vi "Facade.vi"(0 "Data In":T5, 2 "Display State In":T2={"Prompt"="Click to add", "Listbox"=refnum, "events"={"Items Changed"=refnum, "List Changed"=refnum}, "allow move"=FALSE}, 3 "Container State":T4) -> (6 "Data Out":T5, 7 "Display State Out":T2={"Prompt"="Click to add", "Listbox"=refnum, "events"={"Items Changed"=refnum, "List Changed"=refnum}, "allow move"=FALSE}, 8 "Action":T1)   [LabVIEW 2020, in "KListbox.xctl"]
uses:
  KListbox.xctl
  Data.ctl
  <vilib>/_xctls/Container State.ctl
  State.ctl
  Events.ctl
  Event Action.ctl
  <vilib>/_xctls/Action.ctl
  <vilib>/_xctls/XControlSupport.lvlib
panel:
  out "drag from":i32
  in  "Listbox":i32(listbox)
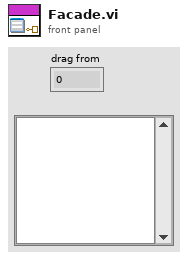
[diagram p1: front panel]
types:
  T1 = typedef "XControlSupport.lvlib/Action.ctl" = cluster{"Data Changed?":bool, "State Changed?":bool, "Action Name":string}
  T2 = typedef "KListbox.xctl/State.ctl" = cluster{"Prompt":string, "Listbox":refnum<vi>, "events":T3, "allow move":bool}
  T3 = typedef "KListbox.xctl/Events.ctl" = cluster{"Items Changed":refnum<user-event>, "List Changed":refnum<user-event>}
  T4 = typedef "XControlSupport.lvlib/Container State.ctl" = cluster{"Indicator?":bool, "Run Mode?":bool, " Refnum":refnum<vi>}
  T5 = typedef "KListbox.xctl/Data.ctl" = cluster{"Row":i32, "Items":string[]}
  T6 = typedef "KListbox.xctl/Event Action.ctl" = enum16{"Select", "Add", "Delete", "Edit"}
  T7 = typedef "LVPoint32TypeDef.ctl" = cluster{"Horizontal":i32, "Vertical":i32}
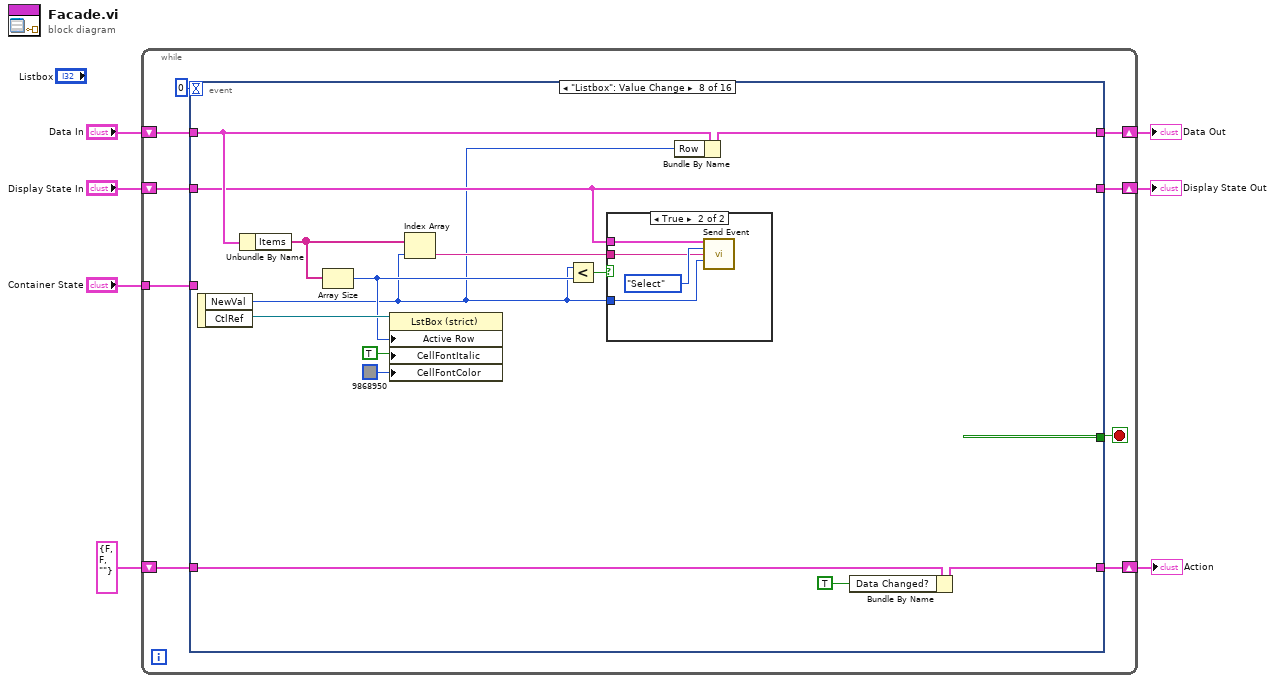
[diagram p0: block diagram]
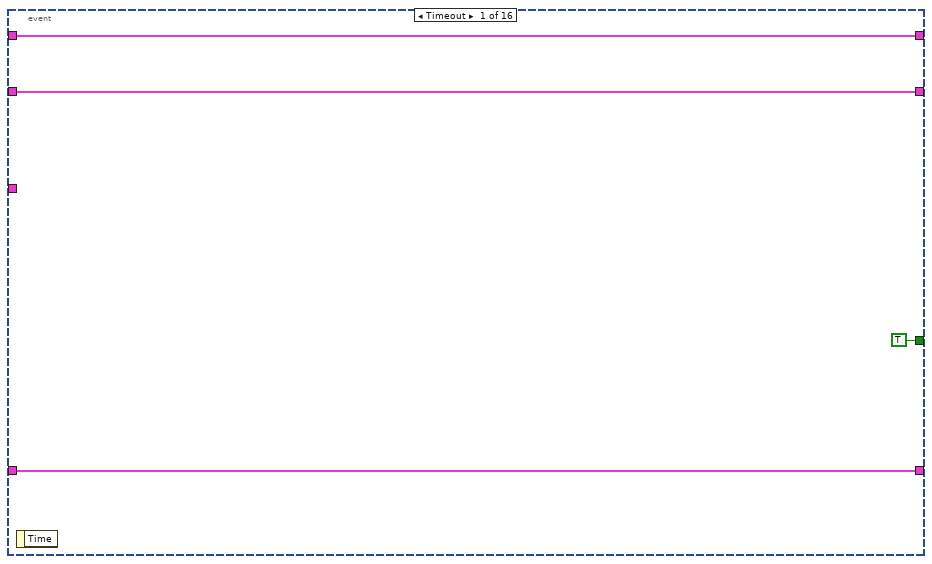
[diagram p2: hidden frame]
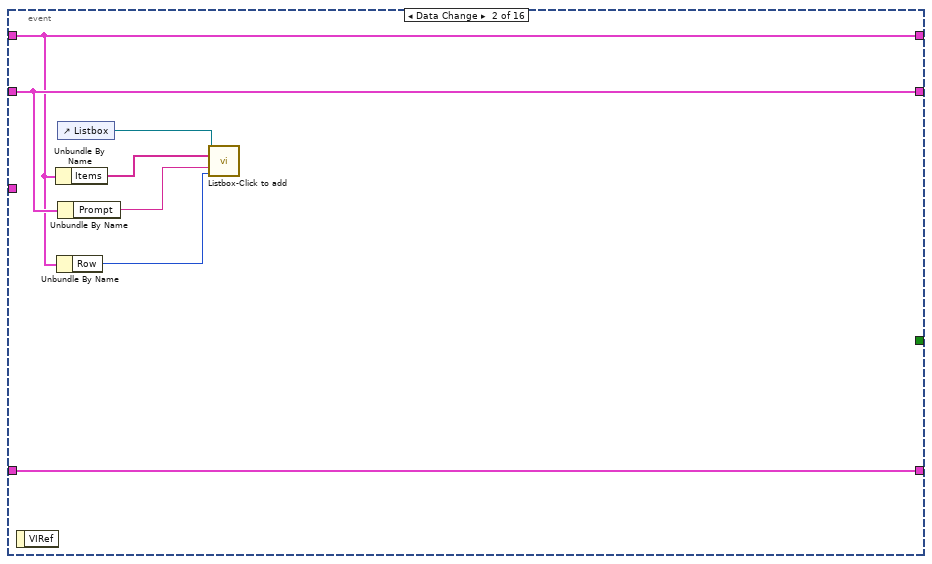
[diagram p3: hidden frame]
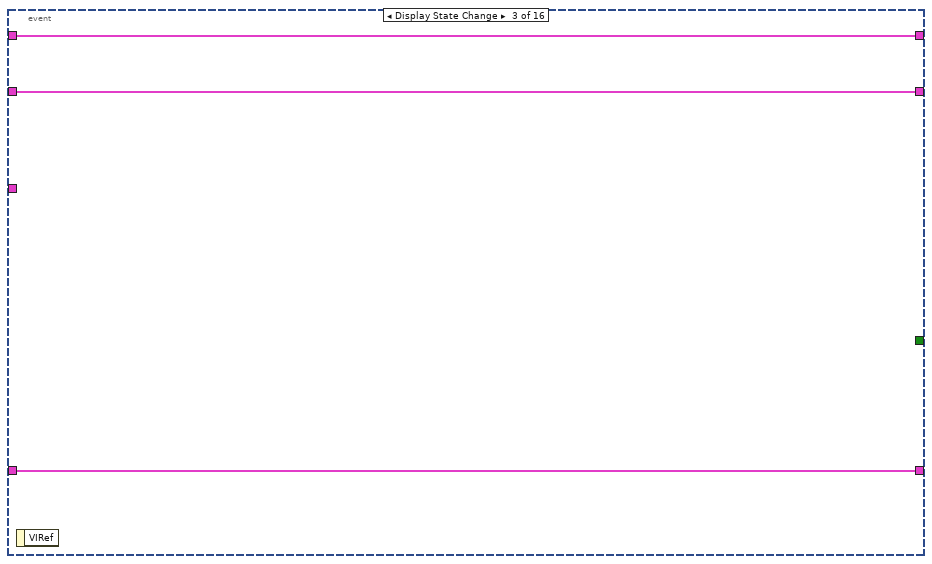
[diagram p4: hidden frame]
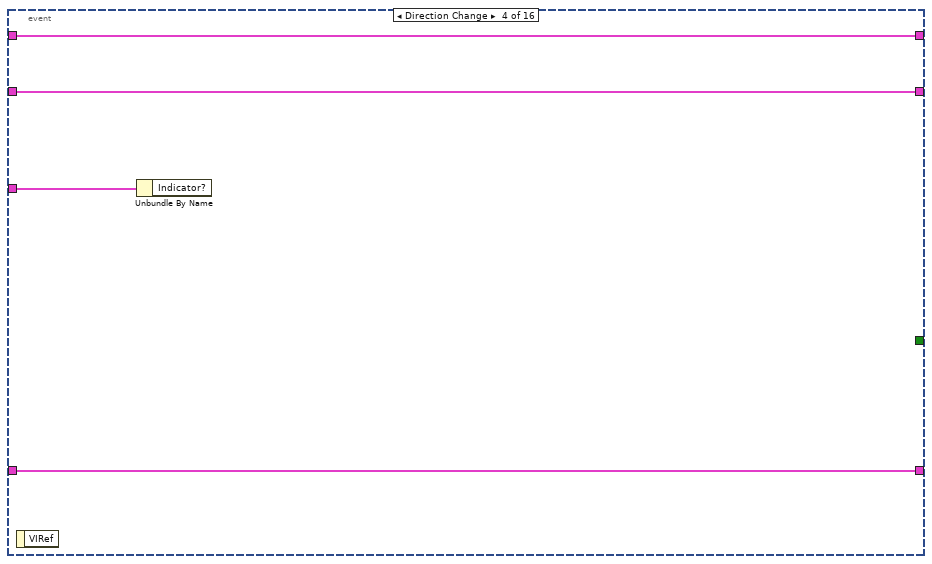
[diagram p5: hidden frame]
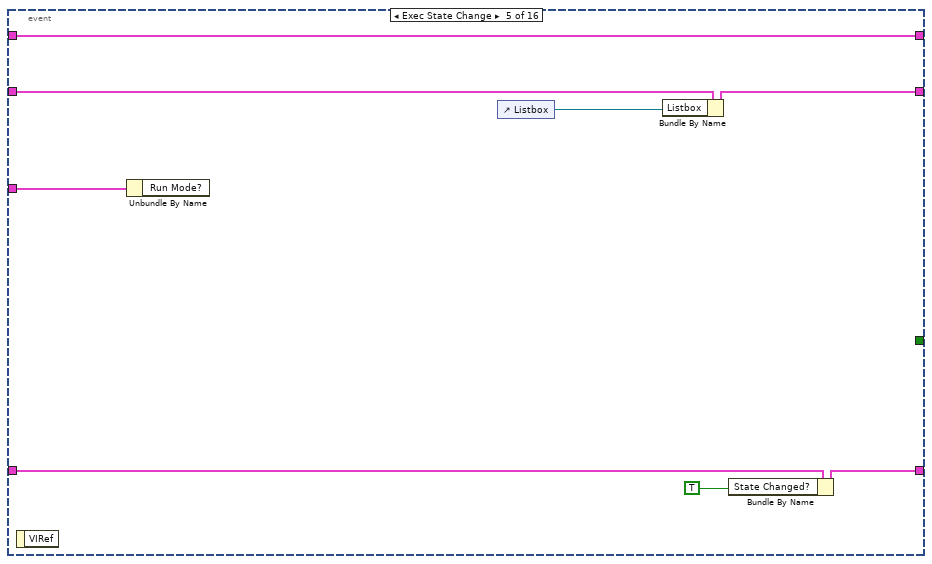
[diagram p6: hidden frame]
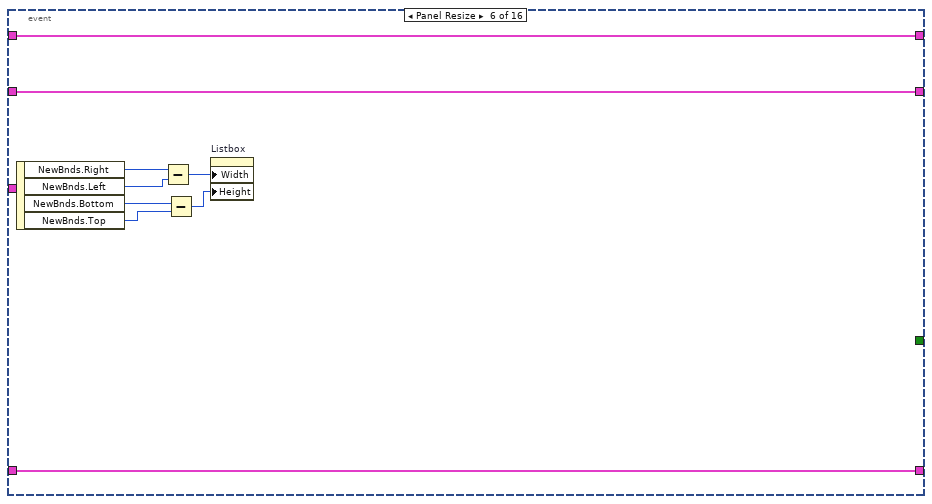
[diagram p7: hidden frame]
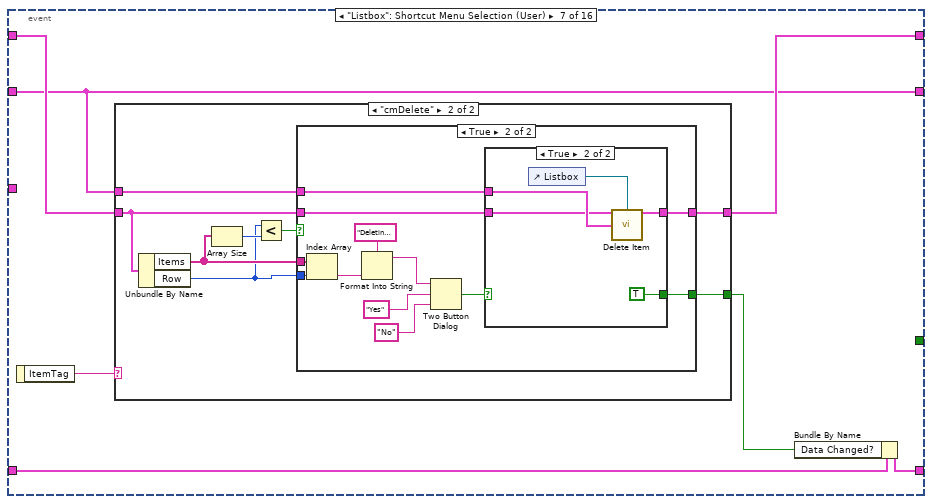
[diagram p8: hidden frame]
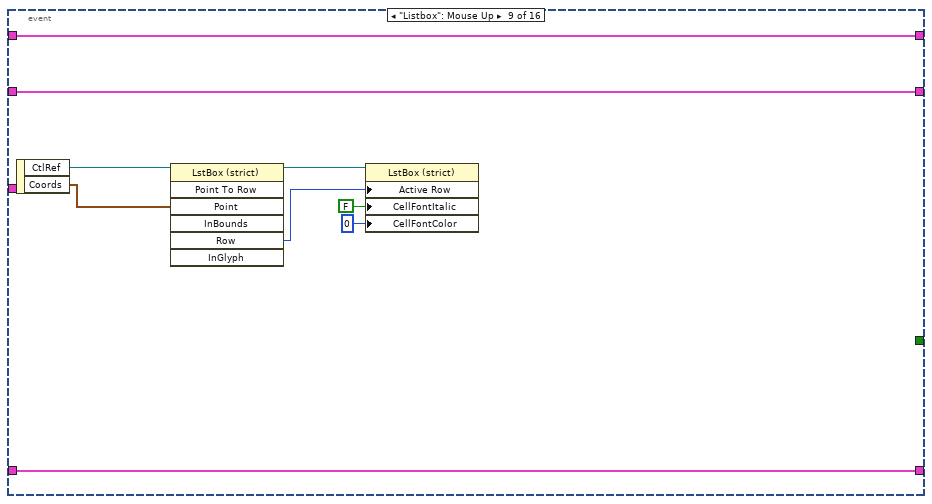
[diagram p13: hidden frame]
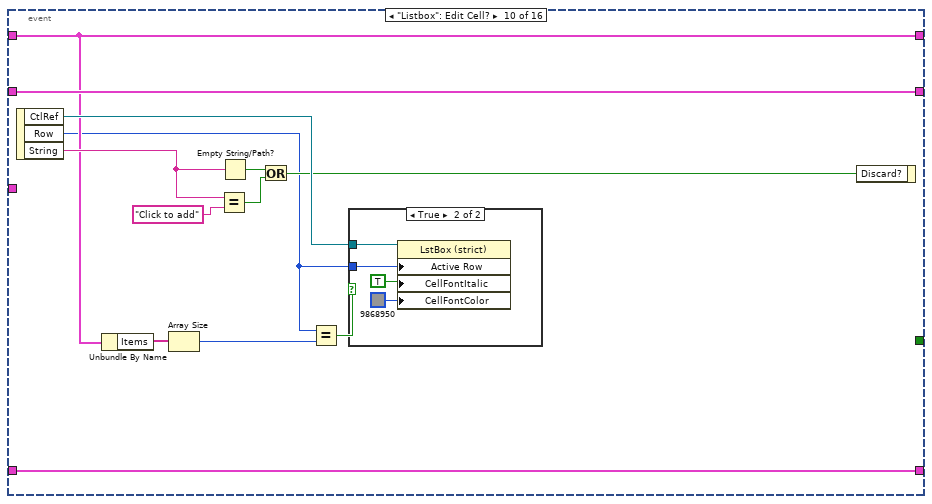
[diagram p14: hidden frame]
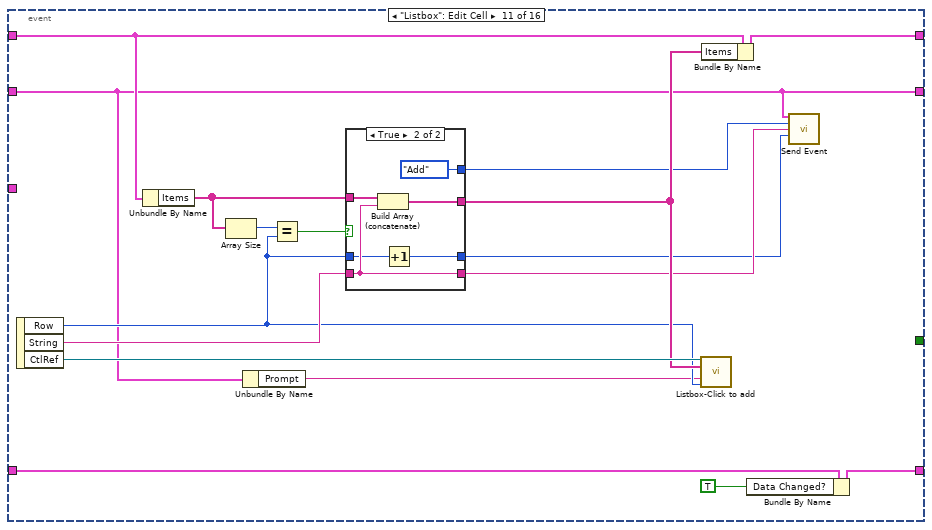
[diagram p16: hidden frame]
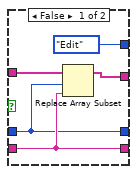
[diagram p17: hidden frame]
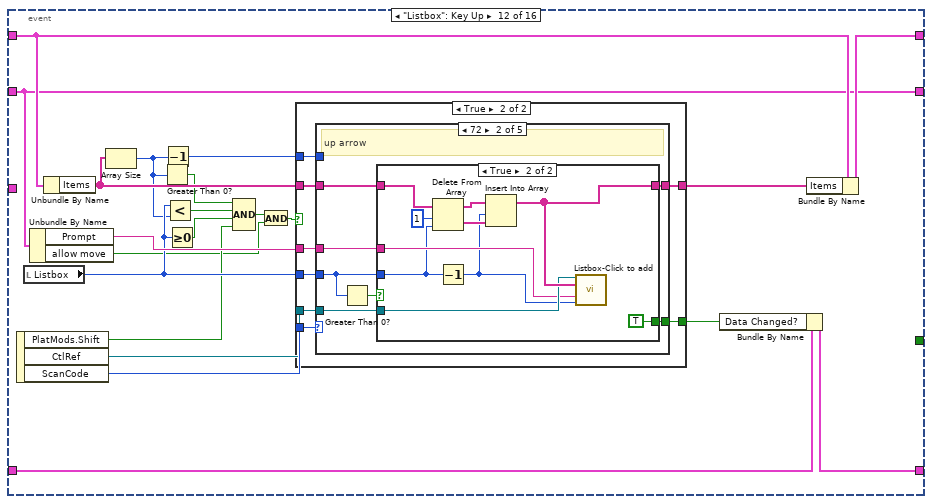
[diagram p18: hidden frame]
diagram:
  n1 = while {
    shift-right: [w15] -> w4
    shift-left: "Display State In" -> [w16]
    tunnel: "Container State" -> [w12]
    shift-right: [w10] -> w7
    shift-left: "Data In" -> [w11]
    shift-right: [w8] -> w2
    shift-left: T1 {"Data Changed?"=FALSE, "State Changed?"=FALSE, "Action Name"=""} ("Action") -> [w9]
    stop <- w14 stop-if-true
    n2 = event shown="[7] \"Listbox\": Value Change" {
      selector: _ -> [_ _ _ _ _ _ _ _ _ _ _ _ _ _ _ _]
      dyn-events: _ -> [_ _ _ _ _ _ _ _ _ _ _ _ _ _ _ _]
      timeout: 0 -> [_ _ _ _ _ _ _ _ _ _ _ _ _ _ _ _]
      tunnel: w16 -> [w18 w26 w30 w33 w41 w51 w53 w92 w113 w126 w134 w171 w251 w255 w265 w268]
      tunnel: [w18 w26 w30 w33 w38 w51 w53 w92 w113 w126 w134 w171 w251 w255 w265 w268] -> w15
      tunnel: [TRUE _ _ _ _ _ _ _ _ _ _ _ _ _ _ _] -> w14
      tunnel: w12 -> [_ _ _ w34 w42 _ _ _ _ _ _ _ _ _ _ _]
      tunnel: w11 -> [w17 w25 w29 w32 w40 w50 w55 w99 w112 w118 w146 w174 w250 w256 w264 w277]
      tunnel: [w17 w25 w29 w32 w40 w50 w54 w95 w112 w118 w141 w173 w250 w256 w264 w274] -> w10
      tunnel: [w19 w27 w28 w31 w36 w49 w56 w94 w111 w125 w140 w178 w249 w261 w263 w272] -> w8
      tunnel: w9 -> [w19 w27 w28 w31 w39 w49 w58 w100 w111 w125 w147 w179 w249 w261 w263 w278]
      event Timeout {
        n3 = event-data() -> ()  [unwired: 1 in, 1 out]
      }
      event Data Change {
        n4 = event-data() -> ()  [unwired: 1 in, 1 out]
        n5 = Unbundle By Name(w25) -> ("Items"=w23:string[])
        n6 = Unbundle By Name(w25) -> ("Row"=w21:i32)
        n7 = control-ref of="Listbox"() -> (w24:refnum<vi>)
        n8 = Unbundle By Name(w26) -> ("Prompt"=w22:string)
        n9 = call "Listbox-Click to add.vi"("ListBox"=w24, "Strings"=w23, "Prompt"=w22, "Row"=w21) -> ()  [unwired: 10 in, 2 out]
      }
      event Display State Change {
        n10 = event-data() -> ()  [unwired: 1 in, 1 out]
      }
      event Direction Change {
        n11 = event-data() -> ()  [unwired: 1 in, 1 out]
        n12 = Unbundle By Name(w34) -> ()  [unwired: 1 out]
      }
      event Exec State Change {
        n13 = event-data() -> ()  [unwired: 1 in, 1 out]
        n14 = Unbundle By Name(w42) -> ()  [unwired: 1 out]
        n15 = control-ref of="Listbox"() -> (w37:refnum<vi>)
        n16 = Bundle By Name(cluster=w41, "Listbox"=w37) -> (w38:T2)
        n17 = Bundle By Name(cluster=w39, "State Changed?"=TRUE) -> (w36:T1)
      }
      event Panel Resize {
        n18 = event-data() -> ("NewBnds.Right"=w48:i16, "NewBnds.Left"=w47:i16, "NewBnds.Bottom"=w46:i16, "NewBnds.Top"=w45:i16)  [unwired: 1 in]
        n19 = Subtract(x=w48, y=w47) -> (x-y=w44:i16)
        n20 = Subtract(x=w46, y=w45) -> (x-y=w43:i16)
        n21 = property on="Listbox" class="LstBox (strict)"("Width"=w44, "Height"=w43) -> ()  [unwired: 2 in, 2 out]
      }
      event "Listbox": Shortcut Menu Selection (User) {
        n22 = event-data() -> ("ItemTag"=w57:string)  [unwired: 1 in]
        n23 = case shown="\"cmDelete\"" w57 {
          tunnel: w55 -> [w59 w65]
          tunnel: [w59 w67] -> w54
          tunnel: w53 -> [_ w66]
          tunnel: [_ w60] -> w52
          frame "", Default {
          }
          frame "cmDelete" {
            n24 = Unbundle By Name(w65) -> ("Items"=w63:string[], "Row"=w62:i32)
            n25 = Array Size(array=w63) -> (size(s)=w64:i32)
            n26 = Less?(x=w62, y=w64) -> (x < y?=w61:bool)
            n27 = case shown="True" w61 {
              tunnel: [w68 w80] -> w67
              tunnel: w66 -> [_ w79]
              tunnel: w65 -> [w68 w78]
              tunnel: w63 -> [_ w71]
              tunnel: w62 -> [_ w70]
              tunnel: [_ w69] -> w60
              frame False {
              }
              frame True {
                n28 = Index Array(array=w71, index=w70) -> (element=w75:string)
                n29 = Format Into String(format string="Deleting '%s' cannot be undone. Are you sure you want to do it?", w75) -> (resulting string=w74:string)  [unwired: 2 in, 1 out]
                n30 = Two Button Dialog(message=w74, 1:"No" ("F button name (\"Cancel\")"), 2:"Yes" ("T button name (\"OK\")")) -> (T button?=w72:bool)
                n31 = case shown="True" w72 {
                  tunnel: [w81 w86] -> w80
                  tunnel: w79 -> [_ w85]
                  tunnel: w78 -> [w81 w84]
                  tunnel: [_ TRUE] -> w69
                  frame False {
                  }
                  frame True {
                    n32 = control-ref of="Listbox"() -> (w82:refnum<vi>)
                    n33 = call "Delete Item.vi"("Data In in"=w84, "LstBox Refnum"=w82, "Display State In"=w85) -> ("Data In out"=w86:T5)  [unwired: 12 in]
                  }
                }
              }
            }
          }
        }
        n34 = Bundle By Name(cluster=w58, "Data Changed?"=w52) -> (w56:T1)
      }
      event "Listbox": Value Change {
        n35 = event-data() -> ("NewVal"=w87:i32, "CtlRef"=w96:refnum<vi>)  [unwired: 1 in]
        n36 = Unbundle By Name(w99) -> ("Items"=w90:string[])
        n37 = Array Size(array=w90) -> (size(s)=w89:i32)
        n38 = property on="Property Node" class="LstBox (strict)"(reference=w96, "Active Row"=w89, "CellFontItalic"=TRUE ("Active Cell:Cell Font:Italic"), "CellFontColor"=u32 9868950) -> ()  [unwired: 1 in, 2 out]
        n39 = Index Array(array=w90, index=w87) -> (element=w88:string)
        n40 = Less?(x=w87, y=w89) -> (x < y?=w91:bool)
        n41 = case shown="True" w91 {
          tunnel: w92 -> [_ w104]
          tunnel: w87 -> [_ w102]
          tunnel: w88 -> [_ w101]
          frame False {
          }
          frame True {
            n42 = call "Send Event.vi"("State"=w104, "action"=Event_Action."Select", "Name"=w101, "Row"=w102) -> ()  [unwired: 10 in, 2 out]
          }
        }
        n43 = Bundle By Name(cluster=w99, "Row"=w87) -> (w95:T5)
        n44 = Bundle By Name(cluster=w100, "Data Changed?"=TRUE) -> (w94:T1)
      }
      event "Listbox": Mouse Up {
        n45 = event-data() -> ("CtlRef"=w106:refnum<vi>, "Coords"=w105:T7)  [unwired: 1 in]
        n46 = invoke on="Invoke Node" class="LstBox (strict)" method="Point To Row"(reference=w106, "Point"=w105) -> (reference out=w107:refnum<vi>, "Row"=w108:i32)  [unwired: 5 in, 5 out]
        n47 = property on="Property Node" class="LstBox (strict)"(reference=w107, "Active Row"=w108, "CellFontItalic"=FALSE ("Active Cell:Cell Font:Italic"), "CellFontColor"=u32 0 ("Active Cell:Cell Font:Color")) -> ()  [unwired: 1 in, 2 out]
      }
      event "Listbox": Edit Cell? {
        n48 = event-data() -> ("CtlRef"=w121:refnum<vi>, "Row"=w116:i32, "String"=w120:string)  [unwired: 1 in]
        n49 = Unbundle By Name(w118) -> ("Items"=w117:string[])
        n50 = Array Size(array=w117) -> (size(s)=w115:i32)
        n51 = Equal?(x=w120, y="Click to add" ("x")) -> (x = y?=w122:bool)
        n52 = Empty String/Path?(string/path=w120) -> (empty?=w123:bool)
        n53 = Or(x=w123, y=w122) -> (x .or. y?=w119:bool)
        n54 = Equal?(x=w116, y=w115) -> (x = y?=w114:bool)
        n55 = case shown="True" w114 {
          tunnel: w121 -> [_ w129]
          tunnel: w116 -> [_ w128]
          frame False {
          }
          frame True {
            n56 = property on="Property Node" class="LstBox (strict)"(reference=w129, "Active Row"=w128, "CellFontItalic"=TRUE ("Active Cell:Cell Font:Italic"), "CellFontColor"=u32 9868950) -> ()  [unwired: 1 in, 2 out]
          }
        }
        n57 = event-data("Discard?"=w119) -> ()  [unwired: 1 in, 1 out]
      }
      event "Listbox": Edit Cell {
        n58 = event-data() -> ("Row"=w136:i32, "String"=w142:string, "CtlRef"=w138:refnum<vi>)  [unwired: 1 in]
        n59 = Unbundle By Name(w146) -> ("Items"=w143:string[])
        n60 = Array Size(array=w143) -> (size(s)=w145:i32)
        n61 = Unbundle By Name(w134) -> ("Prompt"=w135:string)
        n62 = Equal?(x=w145, y=w136) -> (x = y?=w144:bool)
        n63 = case shown="True" w144 {
          tunnel: w143 -> [w152 w158]
          tunnel: w142 -> [w150 w156]
          tunnel: [w151 w157] -> w137
          tunnel: w136 -> [w149 w155]
          tunnel: [w150 w156] -> w133
          tunnel: [w149 w154] -> w132
          tunnel: [Event_Action."Edit" ("action") Event_Action."Add" ("action")] -> w131
          frame False {
            n64 = Replace Array Subset(array=w152, new element=w150, index=w149) -> (w151:string[])
          }
          frame True {
            n65 = Build Array (concatenate)(w158, w156) -> (w157:string[])
            n66 = Increment(x=w155) -> (x+1=w154:i32)
          }
        }
        n67 = call "Listbox-Click to add.vi"("ListBox"=w138, "Strings"=w137, "Prompt"=w135, "Row"=w136) -> ()  [unwired: 10 in, 2 out]
        n68 = Bundle By Name(cluster=w146, "Items"=w137) -> (w141:T5)
        n69 = Bundle By Name(cluster=w147, "Data Changed?"=TRUE) -> (w140:T1)
        n70 = call "Send Event.vi"("State"=w134, "action"=w131, "Name"=w133, "Row"=w132) -> ()  [unwired: 10 in, 2 out]
      }
      event "Listbox": Key Up {
        n71 = event-data() -> ("PlatMods.Shift"=w165:bool, "CtlRef"=w166:refnum<vi>, "ScanCode"=w167:i16)  [unwired: 1 in]
        n72 = local read "Listbox"() -> (w168:i32)
        n73 = Unbundle By Name(w171) -> ("Prompt"=w170:string, "allow move"=w159:bool)
        n74 = Unbundle By Name(w174) -> ("Items"=w177:string[])
        n75 = Array Size(array=w177) -> (size(s)=w163:i32)
        n76 = Greater Than 0?(x=w163) -> (x > 0?=w169:bool)
        n77 = Decrement(x=w163) -> (x-1=w162:i32)
        n78 = Less?(x=w168, y=w163) -> (x < y?=w164:bool)
        n79 = Greater Or Equal To 0?(x=w168) -> (x >= 0?=w176:bool)
        n80 = Compound Arithmetic op=AND(w169, w164, w176, w165) -> (w161:bool)
        n81 = And(x=w161, y=w159) -> (x .and. y?=w160:bool)
        n82 = case shown="True" w160 {
          tunnel: w167 -> [_ w188]
          tunnel: w177 -> [w180 w187]
          tunnel: w168 -> [_ w186]
          tunnel: [w180 w185] -> w172
          tunnel: [_ w184] -> w175
          tunnel: w166 -> [_ w183]
          tunnel: w170 -> [_ w182]
          tunnel: w162 -> [_ w181]
          frame False {
          }
          frame True {
            n83 = case shown="72" w188 {
              tunnel: w187 -> [w189 w196 w215 w235 w242]
              tunnel: w186 -> [_ w190 w209 w230 w237]
              tunnel: [w189 w195 w214 w228 w238] -> w185
              tunnel: [_ w194 w213 TRUE TRUE] -> w184
              tunnel: w183 -> [_ w193 w212 w229 w239]
              tunnel: w182 -> [_ w192 w211 w227 w236]
              tunnel: w181 -> [_ _ w208 _ _]
              frame 0, Default {
              }
              frame 72 {
                # "up arrow"
                n84 = Greater Than 0?(x=w190) -> (x > 0?=w191:bool)
                n85 = case shown="True" w191 {
                  tunnel: w196 -> [w197 w207]
                  tunnel: [w197 w206] -> w195
                  tunnel: [_ TRUE] -> w194
                  tunnel: w193 -> [_ w204]
                  tunnel: w192 -> [_ w203]
                  tunnel: w190 -> [_ w199]
                  frame False {
                  }
                  frame True {
                    n86 = Delete From Array(array=w207, length=1, index=w199) -> (deleted portion=w200:string[], array with subset deleted=w201:string[])
                    n87 = Decrement(x=w199) -> (x-1=w198:i32)
                    n88 = Insert Into Array(array=w201, index=w198, new element=w200) -> (w206:string[])
                    n89 = call "Listbox-Click to add.vi"("ListBox"=w204, "Strings"=w206, "Prompt"=w203, "Row"=w198) -> ()  [unwired: 10 in, 2 out]
                  }
                }
              }
              frame 80 {
                # "down arrow"
                n90 = Less?(x=w209, y=w208) -> (x < y?=w210:bool)
                n91 = case shown="True" w210 {
                  tunnel: w215 -> [w216 w226]
                  tunnel: [w216 w225] -> w214
                  tunnel: [_ TRUE] -> w213
                  tunnel: w212 -> [_ w223]
                  tunnel: w211 -> [_ w222]
                  tunnel: w209 -> [_ w218]
                  frame False {
                  }
                  frame True {
                    n92 = Delete From Array(array=w226, length=1, index=w218) -> (deleted portion=w219:string[], array with subset deleted=w220:string[])
                    n93 = Increment(x=w218) -> (x+1=w217:i32)
                    n94 = Insert Into Array(array=w220, index=w217, new element=w219) -> (w225:string[])
                    n95 = call "Listbox-Click to add.vi"("ListBox"=w223, "Strings"=w225, "Prompt"=w222, "Row"=w217) -> ()  [unwired: 10 in, 2 out]
                  }
                }
              }
              frame 82 {
                # "insert"
                n96 = Format Into String(format string="Item%d", w230) -> (resulting string=w234:string)  [unwired: 2 in, 1 out]
                n97 = Insert Into Array(array=w235, index=w230, new element=w234) -> (w228:string[])
                n98 = call "Listbox-Click to add.vi"("ListBox"=w229, "Strings"=w228, "Prompt"=w227, "Row"=w230) -> ("reference out"=w231:refnum<vi>)  [unwired: 10 in, 1 out]
                n99 = property class="LstBox (strict)"(reference=w231, "EditRow"=w230) -> ()  [unwired: 1 in, 2 out]
              }
              frame 83 {
                # "delete"
                n100 = Delete From Array(array=w242, length=1, index=w237) -> (array with subset deleted=w238:string[])  [unwired: 1 out]
                n101 = call "Listbox-Click to add.vi"("ListBox"=w239, "Strings"=w238, "Prompt"=w236, "Row"=w237) -> ()  [unwired: 10 in, 2 out]
              }
            }
          }
        }
        n102 = Bundle By Name(cluster=w179, "Data Changed?"=w175) -> (w178:T1)
        n103 = Bundle By Name(cluster=w174, "Items"=w172) -> (w173:T5)
      }
      event "Listbox": Key Down? {
        n104 = event-data() -> ("PlatMods.Shift"=w248:bool, "ScanCode"=w246:i16)  [unwired: 1 in]
        n105 = Search 1D Array(1D array=i16[] [72, 80], element=w246) -> (index of element=w245:i32)  [unwired: 1 in]
        n106 = Greater Or Equal To 0?(x=w245) -> (x >= 0?=w244:bool)
        n107 = And(x=w248, y=w244) -> (x .and. y?=w247:bool)
        n108 = event-data("Discard?"=w247) -> ()  [unwired: 1 in, 1 out]
      }
      event "Listbox": Drag Starting? {
        n109 = event-data() -> ()  [unwired: 1 in, 1 out]
        n110 = Unbundle By Name(w256) -> ("Items"=w258:string[])
        n111 = local read "Listbox"() -> (w260:i32)
        n112 = Unbundle By Name(w255) -> ("allow move"=w254:bool)
        n113 = Array Size(array=w258) -> (size(s)=w259:i32)
        n114 = Greater Or Equal?(x=w260, y=w259) -> (x >= y?=w257:bool)
        n115 = Not(x=w254) -> (.not. x?=w253:bool)
        n116 = Or(x=w253, y=w257) -> (x .or. y?=w252:bool)
        n117 = event-data("Discard?"=w252) -> ()  [unwired: 1 in, 1 out]
      }
      event "Listbox": Drag Starting {
        n118 = event-data() -> ()  [unwired: 1 in, 1 out]
        n119 = local read "Listbox"() -> (→"drag from":i32)
      }
      event "Listbox": Drag Ended {
        n120 = event-data() -> ("CtlRef"=w267:refnum<vi>, "Result"=w275:enum16{"Drop Cancel", "Drop Move", "Drop Copy"})  [unwired: 1 in]
        n121 = Unbundle By Name(w268) -> ("Prompt"=w266:string)
        n122 = Unbundle By Name(w277) -> ("Items"=w276:string[])
        n123 = local read "drag from"() -> (w270:i32)
        n124 = local read "Listbox"() -> (w269:i32)
        n125 = case shown="\"Drop Move\"" w275 {
          tunnel: w276 -> [w279 w288]
          tunnel: [w279 w290] -> w273
          tunnel: [_ TRUE] -> w271
          tunnel: w270 -> [_ w292]
          tunnel: w269 -> [_ w282]
          tunnel: w267 -> [_ w291]
          tunnel: w266 -> [_ w289]
          frame "Drop Cancel", Default {
          }
          frame "Drop Move" {
            n126 = Array Size(array=w288) -> (size(s)=w283:i32)
            n127 = Decrement(x=w283) -> (x-1=w281:i32)
            n128 = Max & Min(x=w282, y=w281) -> (min(x,y)=w280:i32)  [unwired: 1 out]
            n129 = Delete From Array(array=w288, length=1, index=w292) -> (deleted portion=w284:string[], array with subset deleted=w285:string[])
            n130 = Insert Into Array(array=w285, index=w280, new element=w284) -> (w290:string[])
            n131 = call "Listbox-Click to add.vi"("ListBox"=w291, "Strings"=w290, "Prompt"=w289, "Row"=w280) -> ()  [unwired: 10 in, 2 out]
          }
        }
        n132 = Bundle By Name(cluster=w278, "Data Changed?"=w271) -> (w272:T1)
        n133 = Bundle By Name(cluster=w277, "Items"=w273) -> (w274:T5)
      }
    }
  }
  "Display State Out" <- w4
  "Data Out" <- w7
  "Action" <- w2
